vi "P2022 TB INCAR_SecuenciaREP.vi"(8 "error in (no error)":errorcluster, 9 "SERIAL MassFlowDevs":T1, 10 "FLOWBUS MassFlowDevs":T1) -> (0 "error out":errorcluster, 1 "Secuencia":string[](array[string]), 2 "Sequence":string, 3 "Secuciclos":string[](array[string]), 11 "Path":path=path "C:/Carboquimica 1/Programas")   [LabVIEW 2013]
uses:
  serialBronkhorst/_s_TablaBronkhorst.ctl
panel:
  in  "Up":bool
  out "Repeticiones":bool
  in  "Finalizar":bool
  in  "Borrar":bool
  in  "Grabar Secuencia":bool
  in  "Cargar Secuencia":bool
  out "Fichero":path
  in  "Linea de comando (doble click)":i32(listbox) caption="Válvulas"
  in  "Secuencia":i32(listbox)=-1
  # "Programador de secuencias"
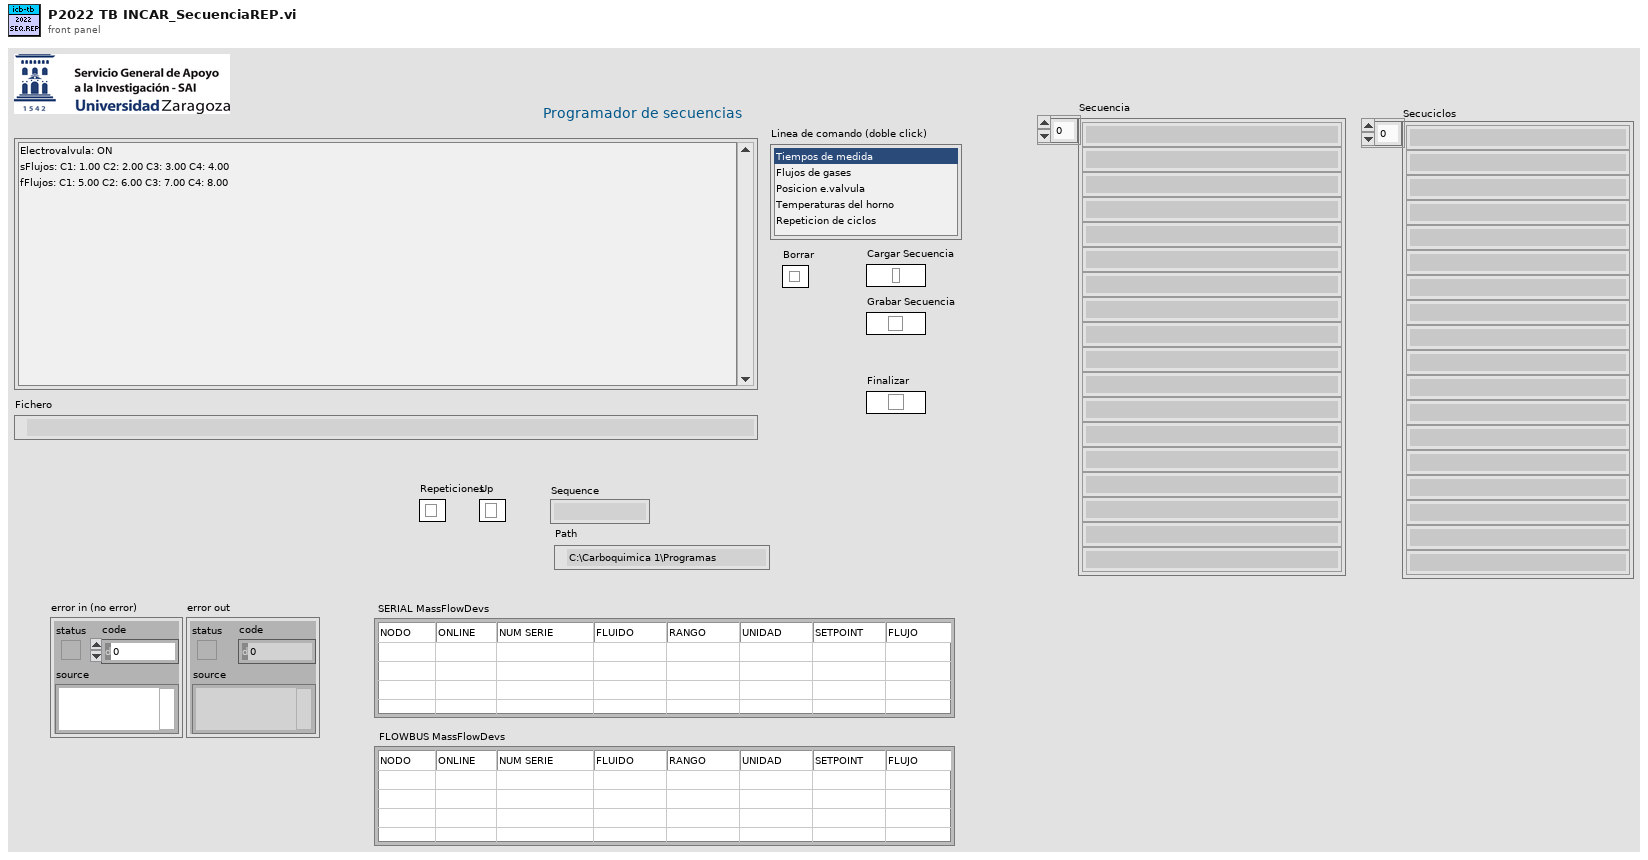
[diagram p1: front panel]
types:
  T1 = typedef "_s_TablaBronkhorst.ctl" = string[][]
  T2 = enum16{"open", "open or create", "create or replace", "create", "open (read only)"}
  T3 = typedef "3xP116.ctl" = cluster{"Ch1":dbl, "Ch2":dbl, "Ch3":dbl}
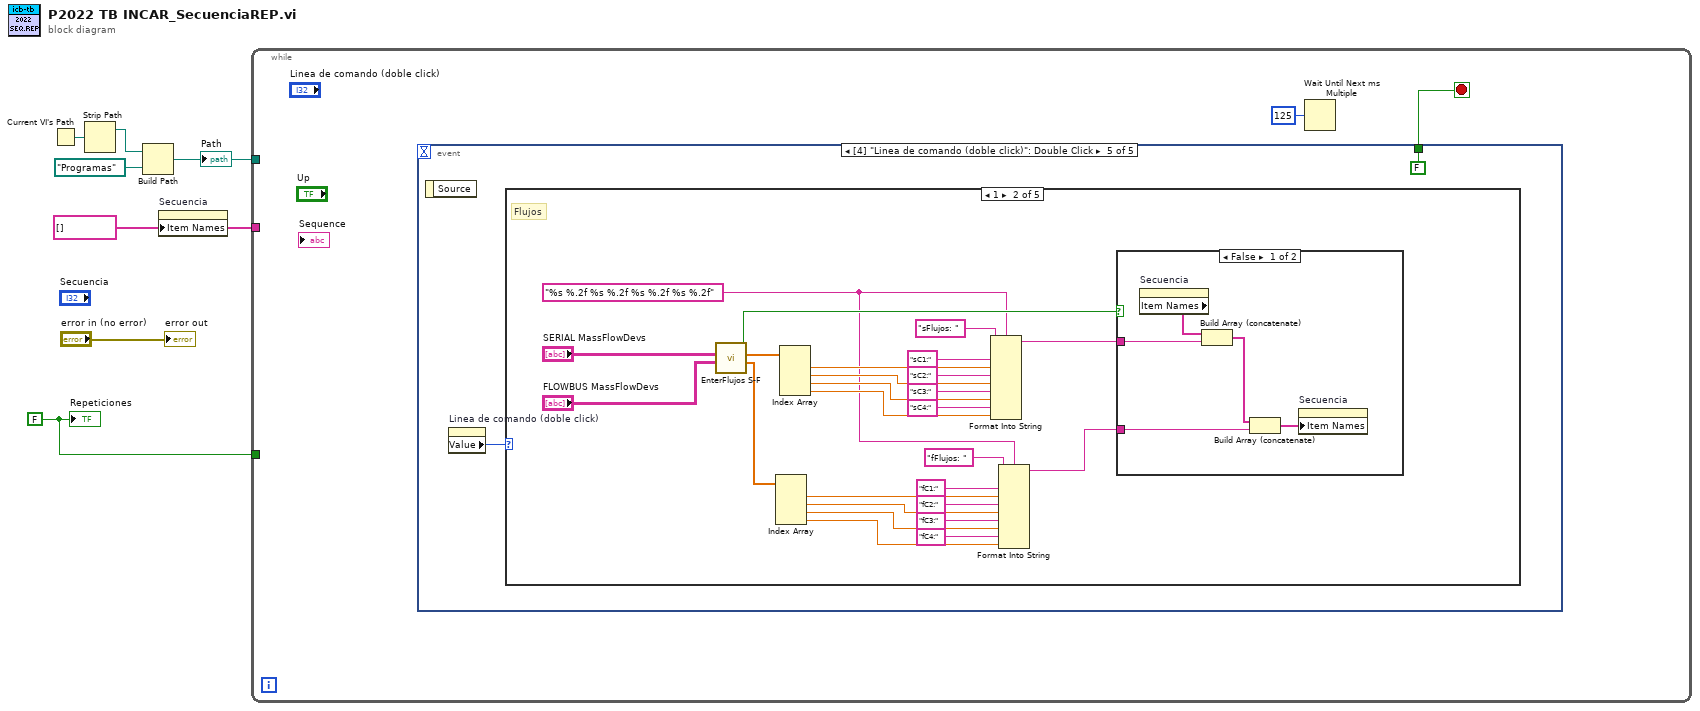
[diagram p0: block diagram]
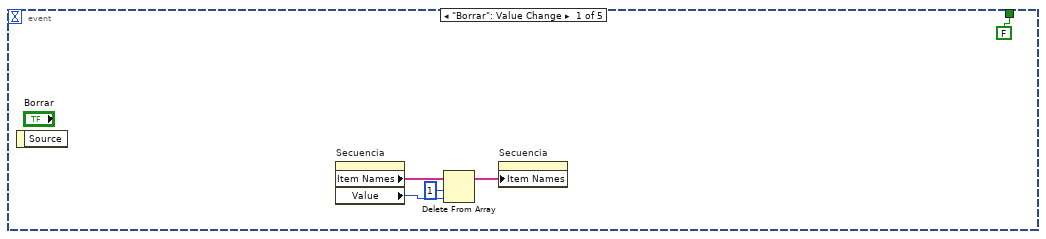
[diagram p2: hidden frame]
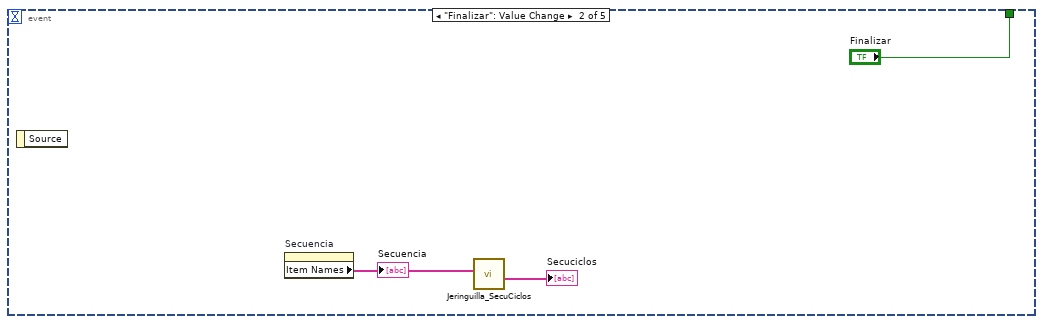
[diagram p3: hidden frame]
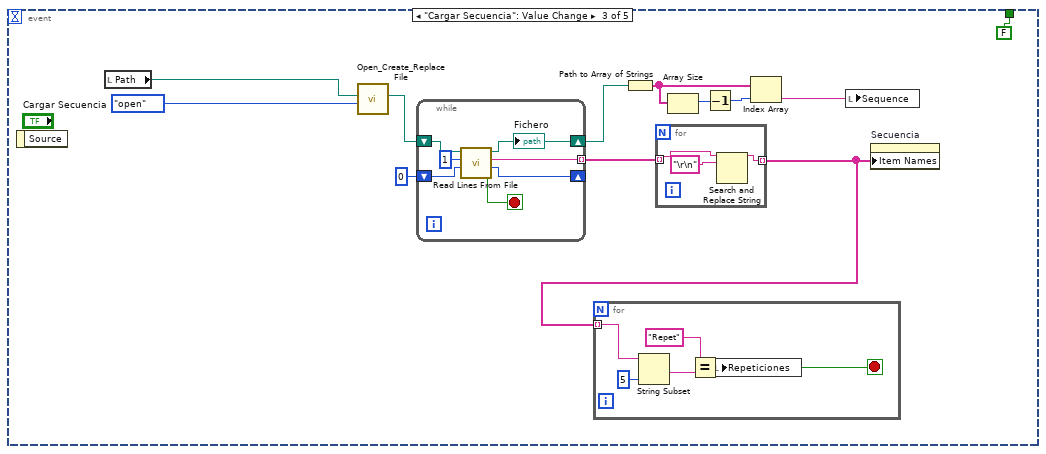
[diagram p4: hidden frame]
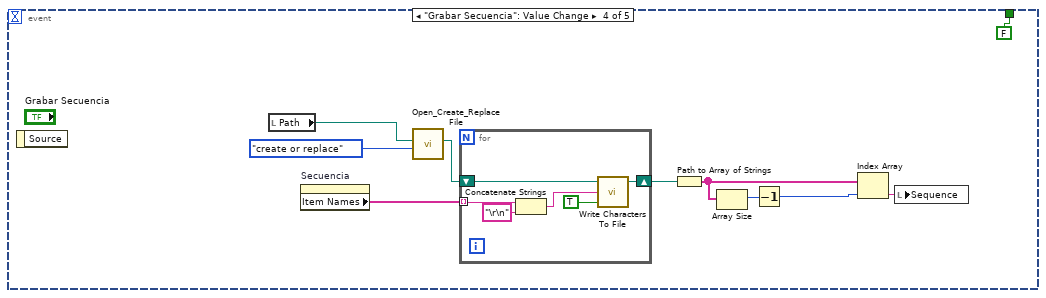
[diagram p5: hidden frame]
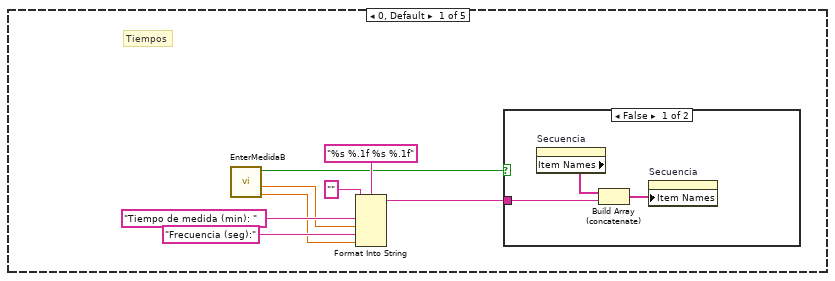
[diagram p6: hidden frame]
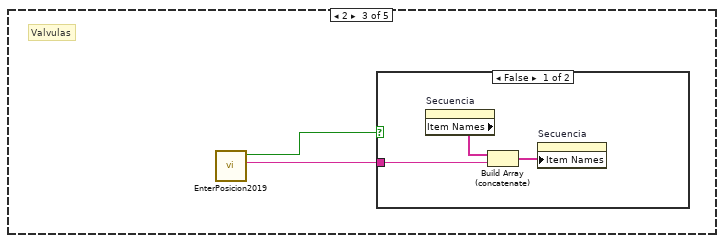
[diagram p9: hidden frame]
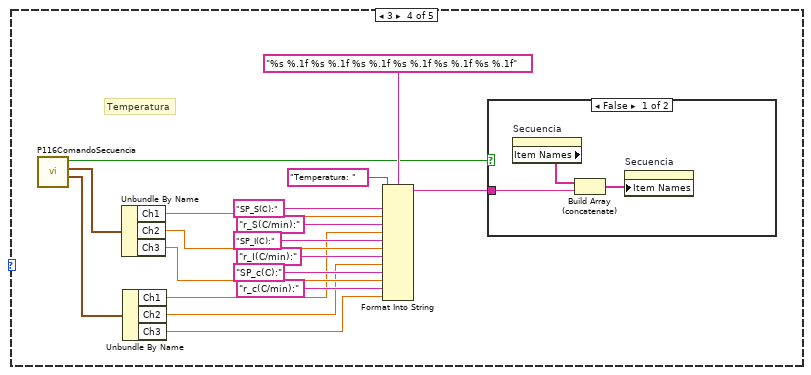
[diagram p11: hidden frame]
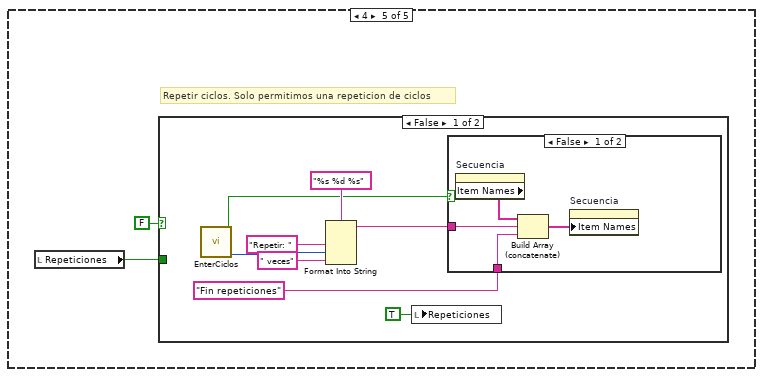
[diagram p13: hidden frame]
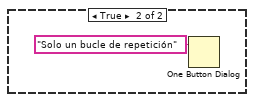
[diagram p15: hidden frame]
diagram:
  w1 = FALSE ("Repeticiones")
  w7 = string[] [] ("Item Names")
  n1 = Current VI's Path() -> (path=w4:path)
  n2 = Strip Path(path=w4) -> (stripped path=w3:path)  [unwired: 1 out]
  n3 = Build Path(base path=w3, name or relative path=path "Programas" ("file path")) -> (appended path=w2:path)
  "Path" <- w2
  n4 = property on="Secuencia" class="LstBox (strict)"("Item Names"=w7) -> ()  [unwired: 2 in, 2 out]
  n5 = while {
    tunnel: w7 -> [_]
    tunnel: w2 -> [_]
    tunnel: w1 -> [_]
    stop <- w8 stop-if-true
    n6 = event shown="[4] \"Linea de comando (doble click)\": Double Click" {
      selector: _ -> [_ _ _ _ _]
      dyn-events: _ -> [_ _ _ _ _]
      timeout: _ -> [_ _ _ _ _]
      tunnel: [FALSE ("Salir") "Finalizar" FALSE ("Salir") FALSE ("Salir") FALSE ("Salir")] -> w8
      event "Borrar": Value Change {
        n7 = event-data() -> ()  [unwired: 1 in, 1 out]
        n8 = property on="Secuencia" class="LstBox (strict)"() -> ("Item Names"=w14:string[], "Value"=w13:i32)  [unwired: 2 in, 2 out]
        n9 = Delete From Array(array=w14, length=1, index=w13) -> (array with subset deleted=w11:string[])  [unwired: 1 out]
        n10 = property on="Secuencia" class="LstBox (strict)"("Item Names"=w11) -> ()  [unwired: 2 in, 2 out]
      }
      event "Finalizar": Value Change {
        n11 = event-data() -> ()  [unwired: 1 in, 1 out]
        n12 = property on="Secuencia" class="LstBox (strict)"() -> ("Item Names"=w16:string[])  [unwired: 2 in, 2 out]
        "Secuencia" <- w16
        n13 = call "Jeringuilla_SecuCiclos.vi"("Secuencia"=w16) -> ("Secuciclos"=→"Secuciclos":string[])  [unwired: 9 in, 1 out]
      }
      event "Cargar Secuencia": Value Change {
        n14 = event-data() -> ()  [unwired: 1 in, 1 out]
        n15 = local read "Path"() -> (w20:path)
        n16 = call <vilib>:"Open_Create_Replace File.vi"("function (open:0)"=T2."open", "start path  (Not A Path)"=w20) -> ("new file path"=w27:path)  [unwired: 6 in, 3 out]
        n17 = while {
          shift-right: [w43] -> w21
          shift-left: w27 -> [w44]
          shift-right: [w40] -> _
          shift-left: 0 ("number of lines (all:-1)") -> [w41]
          tunnel: [w38] -> w26 mode=indexing
          stop <- w39 stop-if-true
          n18 = call <vilib>:"Read Lines From File.vi"("file path (dialog if empty)"=w44, "number of lines (all:-1)"=1, "start of read offset (chars.:0)"=w41) -> ("new file path (Not A Path if cancelled)"=w43:path, "line string"=w38:string, "mark after read (chars.)"=w40:i32, "EOF?"=w39:bool)  [unwired: 3 in]
          "Fichero" <- w43
        }
        n19 = Path to Array of Strings(0:w21) -> (2:w25:string[])  [unwired: 1 out]
        n20 = for {
          tunnel: w26 -> [w36] mode=indexing
          tunnel: [w35] -> w18 mode=indexing
          n21 = Search and Replace String(input string=w36, search string="\r\n") -> (result string=w35:string)  [unwired: 6 in, 3 out]
        }
        n22 = for {
          tunnel: w18 -> [w31] mode=indexing
          stop <- w30 stop-if-true
          n23 = String Subset(string=w31, length (rest)=5 ("length (rest)")) -> (substring=w33:string)  [unwired: 1 in]
          n24 = Equal?(x="Repet" ("input 1"), y=w33) -> (x = y?=w30:bool)
          n25 = local write "Repeticiones"(w30) -> ()
        }
        n26 = Array Size(array=w25) -> (size(s)=w24:i32)
        n27 = Decrement(x=w24) -> (x-1=w23:i32)
        n28 = Index Array(array=w25, index=w23) -> (element=w22:string)
        n29 = local write "Sequence"(w22) -> ()
        n30 = property on="Secuencia" class="LstBox (strict)"("Item Names"=w18) -> ()  [unwired: 2 in, 2 out]
      }
      event "Grabar Secuencia": Value Change {
        n31 = event-data() -> ()  [unwired: 1 in, 1 out]
        n32 = local read "Path"() -> (w46:path)
        n33 = property on="Secuencia" class="LstBox (strict)"() -> ("Item Names"=w54:string[])  [unwired: 2 in, 2 out]
        n34 = call <vilib>:"Open_Create_Replace File.vi"("function (open:0)"=T2."create or replace", "start path  (Not A Path)"=w46) -> ("new file path"=w53:path)  [unwired: 6 in, 3 out]
        n35 = for {
          tunnel: w54 -> [w56] mode=indexing
          shift-right: [w59] -> w48
          shift-left: w53 -> [w60]
          n36 = Concatenate Strings(w56, "\r\n") -> (w55:string)
          n37 = call <vilib>:"Write Characters To File.vi"("append to file? (new file:F)"=TRUE, "character string"=w55, "file path (dialog if empty)"=w60) -> ("new file path (Not A Path if cancelled)"=w59:path)  [unwired: 2 in]
        }
        n38 = Path to Array of Strings(0:w48) -> (2:w51:string[])  [unwired: 1 out]
        n39 = Array Size(array=w51) -> (size(s)=w50:i32)
        n40 = Decrement(x=w50) -> (x-1=w49:i32)
        n41 = Index Array(array=w51, index=w49) -> (element=w47:string)
        n42 = local write "Sequence"(w47) -> ()
      }
      event "Linea de comando (doble click)": Double Click {
        n43 = event-data() -> ()  [unwired: 1 in, 1 out]
        n44 = property on="Linea de comando (doble click)" class="LstBox (strict)"() -> ("Value"=w61:i32)  [unwired: 2 in, 2 out]
        n45 = case shown="1" w61 {
          frame 0, Default {
            # "Tiempos"
            n46 = call "EnterMedidaB.vi"() -> ("Frecuencia (seg)"=w63:dbl, "Tiempo de medida (min)"=w64:dbl, "Cancelled?"=w67:bool)  [unwired: 9 in]
            n47 = Format Into String(format string="%s %.1f %s %.1f", initial string="" ("message"), "Tiempo de medida (min): " ("message"), w64, "Frecuencia (seg):" ("input 1"), w63) -> (resulting string=w68:string)  [unwired: 1 in, 1 out]
            n48 = case shown="False" w67 {
              tunnel: w68 -> [w71 _]
              frame False {
                n49 = property on="Secuencia" class="LstBox (strict)"() -> ("Item Names"=w72:string[])  [unwired: 2 in, 2 out]
                n50 = Build Array (concatenate)(w72, w71) -> (w73:string[])
                n51 = property on="Secuencia" class="LstBox (strict)"("Item Names"=w73) -> ()  [unwired: 2 in, 2 out]
              }
              frame True {
              }
            }
          }
          frame 1 {
            w74 = "%s %.2f %s %.2f %s %.2f %s %.2f" ("format string")
            # "Flujos"
            n52 = call "EnterFlujos S-F.vi"("FLOWBUS MassFlowDevs"="FLOWBUS MassFlowDevs", "SERIAL MassFlowDevs"="SERIAL MassFlowDevs") -> ("%MFCf"=w80:dbl[], "%MFCs"=w81:dbl[], "Cancelled?"=w94:bool)  [unwired: 4 in, 1 out]
            n53 = Index Array(array=w80) -> (element #1=w79:dbl, element #2=w78:dbl, element #3=w77:dbl, element #4=w76:dbl)  [unwired: 4 in]
            n54 = Index Array(array=w81) -> (element #1=w93:dbl, element #2=w92:dbl, element #3=w91:dbl, element #4=w90:dbl)  [unwired: 4 in]
            n55 = Format Into String(format string=w74, initial string="sFlujos: " ("message"), "sC1:" ("input 3"), w93, "sC2:" ("input 3"), w92, "sC3:" ("input 5"), w91, "sC4:" ("input 7"), w90) -> (resulting string=w98:string)  [unwired: 1 in, 1 out]
            n56 = Format Into String(format string=w74, initial string="fFlujos: " ("message"), "fC1:" ("input 3"), w79, "fC2:" ("input 3"), w78, "fC3:" ("input 5"), w77, "fC4:" ("input 7"), w76) -> (resulting string=w75:string)  [unwired: 1 in, 1 out]
            n57 = case shown="False" w94 {
              tunnel: w98 -> [w103 _]
              tunnel: w75 -> [w100 _]
              frame False {
                n58 = property on="Secuencia" class="LstBox (strict)"() -> ("Item Names"=w104:string[])  [unwired: 2 in, 2 out]
                n59 = Build Array (concatenate)(w104, w103) -> (w101:string[])
                n60 = Build Array (concatenate)(w101, w100) -> (w102:string[])
                n61 = property on="Secuencia" class="LstBox (strict)"("Item Names"=w102) -> ()  [unwired: 2 in, 2 out]
              }
              frame True {
              }
            }
          }
          frame 2 {
            # "Valvulas"
            n62 = call "EnterPosicion2019.vi"() -> ("Text"=w105:string, "Cancelled?"=w106:bool)  [unwired: 6 in, 2 out]
            n63 = case shown="False" w106 {
              tunnel: w105 -> [w107 _]
              frame False {
                n64 = property on="Secuencia" class="LstBox (strict)"() -> ("Item Names"=w108:string[])  [unwired: 2 in, 2 out]
                n65 = Build Array (concatenate)(w108, w107) -> (w109:string[])
                n66 = property on="Secuencia" class="LstBox (strict)"("Item Names"=w109) -> ()  [unwired: 2 in, 2 out]
              }
              frame True {
              }
            }
          }
          frame 3 {
            # "Temperatura"
            n67 = call "P116ComandoSecuencia.vi"() -> ("RateSP(C/min) 2"=w117:T3, "NuevoSP(C) 2"=w118:T3, "Cancel 2"=w119:bool)  [unwired: 9 in]
            n68 = Unbundle By Name(w118) -> ("Ch1"=w120:dbl, "Ch2"=w114:dbl, "Ch3"=w113:dbl)
            n69 = Unbundle By Name(w117) -> ("Ch1"=w112:dbl, "Ch2"=w111:dbl, "Ch3"=w110:dbl)
            n70 = Format Into String(format string="%s %.1f %s %.1f %s %.1f %s %.1f %s %.1f %s %.1f", initial string="Temperatura: " ("message"), "SP_S(C):" ("input 1"), w120, "r_S(C/min):" ("input 3"), w112, "SP_I(C):" ("input 1"), w114, "r_I(C/min):" ("input 3"), w111, "SP_c(C):" ("input 1"), w113, "r_c(C/min):" ("input 3"), w110) -> (resulting string=w125:string)  [unwired: 1 in, 1 out]
            n71 = case shown="False" w119 {
              tunnel: w125 -> [w128 _]
              frame False {
                n72 = property on="Secuencia" class="LstBox (strict)"() -> ("Item Names"=w129:string[])  [unwired: 2 in, 2 out]
                n73 = Build Array (concatenate)(w129, w128) -> (w130:string[])
                n74 = property on="Secuencia" class="LstBox (strict)"("Item Names"=w130) -> ()  [unwired: 2 in, 2 out]
              }
              frame True {
              }
            }
          }
          frame 4 {
            # "Repetir ciclos. Solo permitimos una repeticion de ciclos"
            n75 = local read "Repeticiones"() -> (w132:bool)
            n76 = case shown="False" FALSE {
              tunnel: w132 -> [_ _]
              frame False {
                n77 = call "EnterCiclos.vi"() -> ("Ciclos"=w135:i32, "Cancelled?"=w136:bool)  [unwired: 10 in]
                n78 = Format Into String(format string="%s %d %s", "Repetir: " ("input 1"), w135, " veces" ("input 3")) -> (resulting string=w139:string)  [unwired: 2 in, 1 out]
                n79 = local write "Repeticiones"(TRUE ("Repeticiones")) -> ()
                n80 = case shown="False" w136 {
                  tunnel: w139 -> [w142 _]
                  tunnel: "Fin repeticiones" ("input 1") -> [w141 _]
                  frame False {
                    n81 = property on="Secuencia" class="LstBox (strict)"() -> ("Item Names"=w143:string[])  [unwired: 2 in, 2 out]
                    n82 = Build Array (concatenate)(w143, w142, w141) -> (w144:string[])
                    n83 = property on="Secuencia" class="LstBox (strict)"("Item Names"=w144) -> ()  [unwired: 2 in, 2 out]
                  }
                  frame True {
                  }
                }
              }
              frame True {
                n84 = One Button Dialog(message="Solo un bucle de repetición") -> ()  [unwired: 1 in, 1 out]
              }
            }
          }
        }
      }
    }
    n85 = Wait Until Next ms Multiple(millisecond multiple=u32 125) -> ()  [unwired: 1 out]
  }
  "error out" <- "error in (no error)"
  "Repeticiones" <- w1
